vi "AlliGator Logistic Square Gated IRF Characteristics Map.vi"(8 "error in (no error)":errorcluster, 9 "Cursor Names Array":string[](array[string]), 10 "Cursor Positions Array":dbl[](array[numeric]), 11 "AlliGator Internal Variables DVR":refnum<data-value>) -> (0 "error out":errorcluster, 1 "Message":string, 3 "AlliGator Internal Variables DVR":refnum<data-value>)   [LabVIEW 2021, in "AlliGator Scripts.lvlib"]
doc: "Computes the decays of all ROIs and fits them with a logistic square gate model.\n\nSaves the results in an ASCII file."
uses:
  AlliGator Scripts.lvlib
  AlliGator Variables List.ctl
  AlliGator Globals, Variables & Constants.lvlib
  Image/Named ROI Description.ctl
  Image/Image.lvlib
  AlliGator Decay Processing.lvlib
  AlliGator Source Image.lvlib
  <vilib>/vision/Image Controls.llb/IMAQ Image.ctl
  <vilib>/ErrorRing/Error Ring.xnode
  Strings/Strings.lvlib
  Time/Time.lvlib
  AlliGator IRF.lvlib
  Fits/Fit Calculation Method.ctl
  Fits/Fits.lvlib
  Fits/Residual Type.ctl
  Fits/Decay Convolution/Decay Model.ctl
  AlliGator Settings List.ctl
  AlliGator Settings.lvlib
  Fits/Basic Fit Options.ctl
  AlliGator Decay Preprocessing.lvlib
  GUI/GUI.lvlib
  AlliGator Abort.vi
  Fits/Square Pulse/Square Pulse Levels Type.ctl
  Fits/Square Pulse/Square Pulse Options.ctl
  Fits/Non-linear Fitting Algorithm.ctl
  Utilities/Utilities.lvlib
  Fits/IRF(X)PSED/Fit Weights Type.ctl
  Notebook/Notebook.lvlib
  Rich Text Box/Rich Text Box.lvlib
  <vilib>/Utility/error.llb/Error Cluster From Error Code.vi
  <vilib>/Utility/file.llb/Write Delimited Spreadsheet (string).vi
  Variant/Variant to Data/Variant to Data.lvlib
  Fits/Non-linear Fitting Method v2.ctl
  Fits/IRF(X)PSED/Decay Fit Options v2.ctl
  Variant/Variant to Data/Variant to U16.vi
  Phasor/Phasor Reference Series.ctl
  Phasor/Phasor.lvlib
  Phasor/Phasor (g, s).ctl
  Phasor/Calibration Phasor (m, phi).ctl
  AlliGator Data Series Type.ctl
  AlliGator Files.lvlib
  AlliGator Internal Variables v2.ctl
  AlliGator Internal Variables.lvlib
  AlliGator Decay Metadata v3.ctl
  AlliGator Phasor Graph.lvlib
  AlliGator Raw Phasor Plot Data v4.ctl
  AlliGator Baseline Subtraction Method.ctl
  AlliGator Decay Background Subtraction Info.ctl
  Graphs/XY Graph/XY Graph Plot Shift Method.ctl
  Graphs/XY Graph/XY Graph Add-Ons.lvlib
  Graphs/XY Graph/XY Graph Plot Shift Parameters.ctl
  AlliGator Decay Extrapolation Parameters.ctl
  AlliGator FLI Dataset Type.ctl
  Phasor/Phasor Harmonic Data.ctl
  AlliGator Phasor Multi-Harmonic Data.ctl
  AlliGator Phasor Plot.lvlib
  AlliGator Displayed Image.ctl
  Fits/IRF(X)PSED/Decay Fit Parameters & Derived Quantities List.ctl
  Fits/IRF(X)PSED/Decay Fit Parameters In List.ctl
  AlliGator Decay Fit Parameter Constraints 2.ctl
  AlliGator Decay Fit.lvlib
  AlliGator Decay Fit Options & Parameters v2.ctl
  AlliGator Decay Fit Parameter Map.lvlib
  AlliGator Gate Image Set.ctl
  AlliGator Gate Arithmetic.ctl
  AlliGator Dataset Channel.ctl
  AlliGator Dual-Channel Datasets.lvlib
  AlliGator Decay Preprocessing Parameters.ctl
  Phasor/Phasor Standard Deviation Options.ctl
  Phasor/Phasor Calibration Map v2.ctl
  Fits/IRF(X)PSED/MLE Baseline Offset Type.ctl
  AlliGator Parameter Maps Data.ctl
panel:
  # "see the AlliGator License on the block diagram (Ctrl+E or Window:Show Block Diagram)"
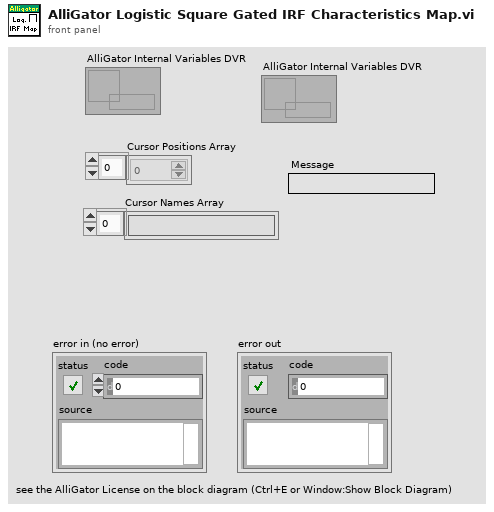
[diagram p1: front panel]
types:
  T1 = typedef "AlliGator Globals, Variables & Constants.lvlib/AlliGator Variables List.ctl" = enum16{"---- GUI ----", "GUI:Initialization Status", "GUI:State Indicators Refnum", "GUI:Original AlliGator Menu Items", "GUI:Current Action Loop State", "GUI:Script in progress", "GUI:Playback", "GUI:Loop Playback", "GUI:Search ROI Used", "GUI:Search ROI", "Decay Graph Max Legend Size", "Intensity Graph Max Legend Size", "Decay Statistics Graph Max Legend Size", "Phasor Graph Max Legend Size", "Phasor Ratio Graph Max Legend Size", "Lifetime Graph Max Legend Size", "---- Files ----", "Files:Export Dataset Frames as Individual Files", "Files:Show Batch Export Help Balloons", "Files:Frames in Dataset", "Files:ptu File Frame Start Indices", "Files:Current Frame in Dataset", "Files:Current Frame Timestamp", "Files:Dataset Loaded", "Files:Dataset Metadata", "Files:Dataset Channel", "Files:Dataset Data Description", "Files:Background Dataset Metadata", "Files:Background Dataset Channel", "Files:Background Dataset Data Description", "Files:Background File Subtraction", "Files:Background File Path", "Files:Background File Pile-up Correction", "Files:Background File Pixel Well Capacity", "Files:Background File Scaling Factor", "Files:Current Dataset Load Settings", "Files:Dataset Path", "Files:ICCD-specific Information", "Files:Macrotime Gate Separation", "------ Python Plugins ------", "Python Plugins:Information", "Python Plugins:Python Session", "Python Plugins:Valid Python Session?", "---- Source Image ----", "Source Image:ROIs", "Source Image:Current ROI", "Source Image:ROI Event Refnum", "X_Source Image Display Range", "X_Source Image Palette Information", "X_Type of Displayed Image", "X_Time Gate Slider", "Source Image:Palette List", "Source Image:Scale", "Source Image:ROI Overlay Color", "Source Image:Overlay to Erase", "Source Image:Is Displayed Image Accumulated", "Source Image:White Light Image Modified", "Source Image:Mask Image Modified", "---- Image Profile Window ----", "Image Profile:Overlay ROI in Source Image", "Image Profile:Window Event Refnum", "Image Profile:IntensityType", "Image Profile:Intensity Average Type", "Image Profile:Intensity-weighted SDV", "Image Profile:Box Profile Type", "Image Profile:Window Open", "Image Profile:Plotted Fit Parameter", "------ Phasor Graph -------", "Phasor Graph:Show Line", "---- Phasor Plot ---", "Phasor Plot:Parameters Changed", "Phasor Plot:FLI Dataset Modified since last Calculation", "Phasor Harmonics Data", "Selected Phasor Harmonics", "Phasor Harmonic Manager Event Refnum", "Phasor Plot:ROIs", "Phasor Plot:Current ROI", "Phasor Plot:ROI Event Refnum", "Phasor Plot:Image Reference Points", "Phasor Plot:Computed", "Phasor Plot:Palette Information", "Phasor Plot:Palette List", "Phasor Plot:Phasor Ratio Palette Information", "Phasor Plot:Phasor Ratio Palette List", "Phasor Plot:Image Scale", "Phasor Plot:Image Overlay to Erase", "Phasor Plot:Image Elements to Update", "Phasor Plot:Current Calculation Parameters", "Phasor Plot:Current Calibration Options", "Phasor Plot:Reset Cumulated Phasor Plot", "Phasor Plot:Reference 1", "Phasor Plot:Lifetime Reference 1", "Phasor Plot:Reference 1 Frequency", "Phasor Plot:Reference 2", "Phasor Plot:Lifetime Reference 2", "Phasor Plot:Reference 2 Frequency", "---- Decay Analysis ----", "Number of Selected Decays to Fit", "LS Fit Results", "LAR Fit Results", "BS Fit Results", "Last Decay Max - Min", "Best Fit Parameters", "Best Fit Parameter Names", "Actual Size X", "Actual Size Y", "Binning X", "Binning Y", "Actual # Gates", "Dataset Number", "Gates to...", "Gates Skipped", "Gates to keep", "Gate Step", "Gate Separation", "Reversed Gates", "Pile-up Correction", "Pixel Well Capacity", "Background Subtracted", "Background Subtraction Method", "Background Definition Range", "Background File (deprecated)", "Number of Dataset Accumulated", "Array of Accumulated Dataset Paths", "Do Averaged Datasets", "Destination File Path", "Process Plot Target", "Use 1/D as Phasor Frequency", "---- Decay Fit Parameter Map -----", "Decay Fit Parameter Map:Palette Information", "Decay Fit Parameter Map:Palette List", "------- Local Decay Window ---------", "Local Decay Graph Window:Event Refnum", "Local Decay Graph Window:Use normalized IRF for convolution", "----- Miscellaneous ----", "Misc:Skippable Dialog Windows Status"}
  T2 = typedef "IMAQ Image.ctl" = refnum<image>
  T3 = typedef "Fits.lvlib/Square Pulse Options.ctl" = cluster{"Method":T4, "# Bins":i32, "Threshold %":dbl, "Center on Midpoint":bool, "Smoothen Plot":bool}
  T4 = typedef "Fits.lvlib/Square Pulse Levels Type.ctl" = enum16{"Mode", "Mean"}
  T5 = typedef "AlliGator Settings.lvlib/AlliGator Settings List.ctl" = enum16{"GUI:Visible Settings Tab", "GUI:Last Run Version", "Source Image:Use Image Histogram for Contrast", "Source Image:Low Count Pixels Rejection Options", "Source Image:High Count Pixels Rejection Options", "Source Image:Use Image Brightness", "Source Image:Blend Overlay with Image Background", "Source Image:Use Fixed ROI Diameter", "Source Image:ROI Diameter", "Source Image:ROI Center Color", "Source Image:Peak Threshold", "Source Image:Intensity Threshold", "Source Image:Image Binning Options", "Source Image:Image Smoothing Options", "Source Image:Image Histogram Active", "Source Image:Invert Binary Mask", "Source Image:Hot Pixel Removal", "Source Image:Overlay Analyzed ROI Center", "Source Image:Auto-Adjust Contrast", "Source Image:Histogram Lower Percentile", "Source Image:Histogram Upper Percentile", "Source Image:Save Source Image", "Source Image:Scale Bar Options", "Source Image:Image Resolution (Pixel Size)", "Source Image:Flatfield Correction", "Source Image:Show Dead Left Columns Correction", "Source Image:Dead Left Columns Correction", "Source Image:Image Pre-Processing Operations Order", "Data Information:Gate Width", "Data Information:Nanotime Gate Separation", "Data Information:Macrotime Gate Separation", "Data Information:Gate Step", "Data Information:# Gates", "Data Information:Gate Image Exposure", "Data Information:Gate Image Integration", "Data Information:Gates to Skip", "Data Information:Gates to Keep", "Data Information:Define Gates to", "Data Information:Channel Name", "Data Information:Available Channel Names", "Data Information:Channel Arithmetic", "Data Information:Background File Subtraction", "Data Information:Background File", "Data Information:Background Scaling Factor", "Data Information:Background Pile-up Correction", "Data Information:Background Pixel Well Capacity", "Data Information:Laser Period", "Data Information:SYNC Period", "Data Information:Pile-up Correction", "Data Information:Pixel Well Capacity", "Data Information:Dataset Scaling Factor", "Fluorescence Decay_Decay Pre-Processing:Reverse Gates", "Fluorescence Decay_Decay Pre-Processing:Verbose Decay Pre-Processing", "Fluorescence Decay_Decay Pre-Processing:Use Decay Pre-Processing", "Fluorescence Decay_Decay Pre-Processing:Background Subtraction", "Fluorescence Decay_Decay Pre-Processing:Background Definition Range", "Fluorescence Decay_Decay Pre-Processing:Baseline Subtraction Method", "Fluorescence Decay_Decay Pre-Processing:Decay Pre-Processing Operations Order", "Fluorescence Decay_Decay Pre-Processing:Smoothing Parameter", "Fluorescence Decay_Decay Pre-Processing:Shift Decay", "Fluorescence Decay_Decay Pre-Processing:Decay Shift Parameters", "Fluorescence Decay_Decay Pre-Processing:Fold Decay", "Fluorescence Decay_Decay Pre-Processing:# Folds", "Fluorescence Decay_Decay Pre-Processing:1-Normalize Decay", "Fluorescence Decay_Decay Pre-Processing:[0-1]-Normalize Decay", "Fluorescence Decay_Decay Pre-Processing:Smoothen Decay", "Fluorescence Decay_Decay Pre-Processing:Extrapolate Decay", "Fluorescence Decay_Decay Pre-Processing:Use Periodicity", "Fluorescence Decay_Decay Pre-Processing:Use Cursors", "Fluorescence Decay_Decay Pre-Processing:Tail Fraction", "Fluorescence Decay_Decay Pre-Processing:Head Fraction", "Fluorescence Decay_Decay Pre-Processing:Additional Points", "Fluorescence Decay_Decay Pre-Processing:Straighten Decay", "Fluorescence Decay_Decay Pre-Processing:Constant Background", "Fluorescence Decay_Decay Pre-Processing:Pixel-Normalize Decay", "Fluorescence Decay_Advanced Analysis:Extract IRF instead of Decay", "Fluorescence Decay_Advanced Analysis:IRF Extraction Options", "Fluorescence Decay_Advanced Analysis:IRF Optimization Options", "Fluorescence Decay_Advanced Analysis:Square Pulse Options", "Fluorescence Decay_Advanced Analysis:IRF Order", "Fluorescence Decay_Advanced Analysis:IRF Time Constants", "Fluorescence Decay_Advanced Analysis:Wavelet Analysis Options", "Fluorescence Decay_Advanced Analysis:Average Lifetime Options", "Fluorescence Decay_Fit Options:Fit Options", "Fluorescence Decay_Fit Options:Use Legacy Fitting Approach", "Fluorescence Decay_Fit Options:Use Data Information Laser Period", "Fluorescence Decay_Fit Parameters:Displayed Fit Parameters", "Fluorescence Decay_Fit Parameters:Fit Parameter Constraints", "Fluorescence Decay_Fit Parameters:Export Tabulated Results", "Fluorescence Decay_Fit Parameters:MLE Baseline Offset Type", "Fluorescence Decay_Fit Parameters:MLE Baseline Offset", "Fluorescence Decay_Fit Parameters:Guess Parameter Names", "Fluorescence Decay_Fit Parameters:Guess Parameter Values", "Fluorescence Decay_Fit Parameters:Guess Parameters Options", "Fluorescence Decay_Styles:Show Last Decay Only", "Fluorescence Decay_Styles:Decay Graph Color Array", "Fluorescence Decay:Decay Graph Active", "Fluorescence Decay Statistics:Min Peak Value", "Fluorescence Decay Statistics:Reject Low Decay Peak Pixels", "Fluorescence Decay Statistics:Reject High Decay Peak Pixels", "Fluorescence Decay Statistics:Max Peak Value", "Time Traces:Use File Timestamp", "Time Traces:Time Step", "Time Traces:Use Intensity Correction File", "Time Traces:Intensity Correction File", "Phasor Plot:Phasor Plot Smoothing Options", "Phasor Plot:Phasor Plot Size", "Phasor Plot:Phasor Plot Graphics Options", "Phasor Plot:Cumulative Phasor Plot", "Phasor Plot:Use Phasor Brightness", "Phasor Plot:Blend Overlay with Phasor Background", "Phasor Plot:Save Phasor Plot", "Phasor Plot:Show References", "Phasor Plot:Phasor Ratio Decay Range", "Phasor Plot:Exponential Fading", "Phasor Plot:Phasor Ratio Reference Colors", "Phasor Plot:Reference Radius", "Phasor Plot:Show Color Map Vertices", "Phasor Plot:Phasor Plot Active", "Phasor Plot:Phasor Ratio Color Map Type", "Phasor Plot:Phasor Ratio Color Map", "Phasor Plot:Phasor Ratio Display Range", "Phasor Plot:Selected Image ROI(s)", "Phasor Plot:All Image ROIs", "Phasor Plot:Selected Phasor Plot ROI(s)", "Phasor Plot:All Phasor Plot ROIs", "Phasor Plot:Phasor Ratio Color-Coded Quantity", "Phasor Plot:Store Phasor Harmonics", "Phasor Plot:Draw Reference Segment", "Phasor Plot:User-Defined Quantity", "Phasor Graph:Phasor Frequency", "Phasor Graph:Phasor Ratio Type", "Phasor Graph:Pixel-level Phasor Computation", "Phasor Graph:Save Phasor Graph", "Phasor Graph:Phasor Graph Active", "Phasor Graph:Phasor SDV Options", "Phasor Calibration:Use Backup Calibration if needed", "Phasor Graph:Define Shortest Lifetime as", "Phasor Calibration:Backup Calibration Type", "Phasor Calibration:Calibration Type", "Phasor Calibration:Calibration Lifetime", "Phasor Calibration:Calibration Map Algorithm", "Single-Exponential Phasor Locus (SEPL):Gate Parameters", "Single-Exponential Phasor Locus (SEPL):User-defined Gate", "Single-Exponential Phasor Locus (SEPL):User-defined IRF", "Single-Exponential Phasor Locus (SEPL):Phasor Parameters", "Single-Exponential Phasor Locus (SEPL):Decay & IRF Parameters", "Single-Exponential Phasor Locus (SEPL):Display Parameters", "Lifetime Analysis:Decay Analysis Parameters", "Lifetime Analysis:Lifetime Map Active", "Plugins:Python Settings", "Miscellaneous:Verbose Mode", "Miscellaneous:Beep after Script", "Miscellaneous:Saved Image File Format", "Miscellaneous:Exported Gate Image Settings", "Miscellaneous:Include Loading in Timing", "Miscellaneous:Verbose Settings Mode", "Miscellaneous:Histogram Options", "Miscellaneous:Beep on Error", "Miscellaneous:# Logical Processors Used", "Miscellaneous:ROI Description Max Characters", "Miscellaneous:Verbose Error Mode", "Miscellaneous:Transparent Mask Color"}
  T6 = typedef "Fits.lvlib/Basic Fit Options.ctl" = cluster{"Fitting Method":T7, "Weighted Fit":bool, "Residual Type":T8, "Compute Parameter Uncertainties":bool, "Fitting Algorithm":T9}
  T7 = typedef "Fits.lvlib/Non-linear Fitting Method v2.ctl" = enum16{"Least Square", "Least Absolute Residual", "Bisquare", "MLE", "-", "Best of All"}
  T8 = typedef "Fits.lvlib/Residual Type.ctl" = enum16{"Standard", "Normalized", "Reduced"}
  T9 = typedef "Fits.lvlib/Non-linear Fitting Algorithm.ctl" = enum16{"Levenberg-Marquardt", "Trust-Region Dogleg"}
  T10 = typedef "Fits.lvlib/Decay Fit Options v2.ctl" = cluster{"Show Fit Residuals":bool, "Fit Model":T11, "Residual Type":T8, "Max Decay Percentile":dbl, "Min Decay Percentile":dbl, "Show Full Decay":bool, "Weights":T12, "Fitting Method":T7, "Compute Parameter Uncertainties":bool, "Periodic Boundaries":bool, "Model Calculation":T13, "Period":dbl[unit], "Termination Criteria":cluster{"Max Iterations":i32, "Max Function Calls":i32, "Max Time":dbl[unit], "Function Tolerance":dbl, "Parameter Tolerance":dbl, "Gradient Tolerance":dbl, "Min Lambda":dbl, "Max Lambda":dbl, "Initial Tick Count":u32}, "Offset Resolution":dbl[unit], "Use Local IRF":bool, "Fitting Algorithm":T9}
  T11 = typedef "Fits.lvlib/Decay Model.ctl" = enum16{"1-Exponential", "2-Exponentials"}
  T12 = typedef "Fits.lvlib/Fit Weights Type.ctl" = enum16{"Unweighted", "1/Variance", "Best of All"}
  T13 = typedef "Fits.lvlib/Fit Calculation Method.ctl" = enum16{"Simulation", "Convolution", "Integration"}
  T14 = typedef "Image.lvlib/Named ROI Description.ctl" = cluster{"ROI Descriptor":T15, "ROI Name":string, "Overlay Color":u32}
  T15 = typedef "ROI Descriptor" = cluster{"Global Rectangle":i32[], "Contours":cluster{"ID":enum32{"External", "Internal"}, "Type":u32, "Coordinates":i32[]}[]}
  T16 = typedef "AlliGator Internal Variables.lvlib/AlliGator Internal Variables v2.ctl" = cluster{"Displayed Image":T2, "White Light Image":T2, "Mask Image":T2, "ROI Mask Image":T2, "Current Dataset Images 1":T17, "Background Dataset Images 1":T17, "Current Dataset Images 2":T17, "Background Dataset Images 2":T17, "Current Dataset Arithmetic Images":T17, "Accumulated Dataset Images 1":T17, "Accumulated Dataset Images 2":T17, "Accumulated Dataset Arithmetic Images":T17, "Phasor Plot Image":T2, "Decay Fit Parameter Map Image":T2, "Single Data Point Path":path, "White Light Image Path":path, "Mask Image Path":path, "Time-Series Folder":path, "[Time-Series Paths]":path[], "Current Dataset":i32, "Single Dataset Type":T18, "Current Folder":string, "AlliGator Data Series Type":T19, "# Datasets":i32, "Dual-Channel Dataset":bool, "Selected Channel Name":string, "Dataset Channel":T20, "Channel Arithmetic":T21, "Dual-Channel Background Dataset":bool, "Background Channel":T20, "Dual-Channel Accumulated Dataset":bool, "Start Time":dbl, "[Time-Series Timestamps]":dbl[], "[Intensity Corrections]":dbl[], "Time Series Script":bool, "Type of Displayed Image":T22, "Gate Image Slide":u16, "# Gates":i32, "ROIs":T14[], "ROI Decay":cluster{"t Array":dbl[], "I Array":dbl[]}, "Valid Decay":bool, "Decay  Metadata":T23, "Reference Decay Plot Name":string, "Reference Decay":cluster{"t Array":dbl[], "I Array":dbl[]}, "Decay Shift Plot":cluster{"Time Stamps":dbl[], "Decay Shifts":dbl[]}, "[Decays Max Values]":sgl[], "[Decays Min Values]":sgl[], "Calibration Phasor":T29, "Calibration Phasor Series":T30, "Phasor Calibration Map":T31, "Calibration Map MD5 Digest":string, "Last Raw Phasor":T32, "Last Calibrated Phasor":T32, "Last Calibrated Phasor SDV":T32, "Phasor Graph:Phasor Plot":cluster{"g Array":dbl[], "s Array":dbl[]}, "Phasor Graph:Phasor SDV Plot":cluster{"g Array":dbl[], "s Array":dbl[]}, "[Phasor Graph:Raw Phasor Plots]":T33[], "Phasor Plot locked to Ref 1":i32, "[Phasor Plot(s) locked to Ref 1]":i32[], "[Phasor Plot(s) locked to Ref 2]":i32[], "[Pixel Phasors]":T32[], "[[Sum Image]]":dbl[][], "[[CSG Phasors]]":csg[][], "[[Valid Pixel?]]":bool[][], "I/m/phi Dataset":cluster{"I/m/phi Dataset?":bool, "Base Frequency":dbl[unit], "Harmonic Orders":u8[]}, "Multi Phasor Plot Data":T35, "Decay Fit Options & Parameters":T37, "Fit Options: Decay Preprocessing Parameters":T41, "Fit Options: Reference Decay":cluster{"t Array":dbl[], "I Array":dbl[]}, "Is Full Image Parameters Map":bool, "Is Single-Pixels Parameters Map":bool, "NLSF Parameters Map X Resolution":i32, "NLSF Parameters Map Y Resolution":i32, "[Single Decay Fit Parameters]":dbl[], "Fit Model":T11, "[[Multiple Decays Fit Parameters]]":dbl[][], "[[Multiple Decays Fit Parameter SDVs]]":dbl[][], "[[IRFs]]":dbl[][], "IRF Array Time Axis":dbl[], "Decay Array Time Axis":dbl[], "[Decay Fit Parameter Names]":T42[], "[[Phasor Ratios]]":dbl[][], "[[Average Lifetimes]]":dbl[][], "Amplitude Weighted Average Lifetime":bool, "[Decay Sum]":dbl[], "Parameter Maps":T43[], "[[User-defined Quantities]]":dbl[][], "User-defined Quantity":string}
  T17 = typedef "AlliGator Internal Variables.lvlib/AlliGator Gate Image Set.ctl" = cluster{"SGL Image Max":T2, "SGL Image Sum":T2, "SGL Gate Images":T2[], "SGL Image Min":T2}
  T18 = typedef "AlliGator Files.lvlib/AlliGator FLI Dataset Type.ctl" = enum16{"HDF5 FLI Dataset", "Gate Image Folder", ".sdt FLI Dataset (Becker & Hickl)", ".ptu FLI Dataset (PicoQuant)", "SS1 FLI Dataset", "SS2 FLI Dataset", "I/m/phi Dataset", ".bin FLI Dataset (PicoQuant Binned)", ".bin FLI Dataset (Piccolo Binned)"}
  T19 = typedef "AlliGator Files.lvlib/AlliGator Data Series Type.ctl" = enum16{"Not a Supported Series", "Gate Images Folder Series", "SwissSPAD 2 Dataset Series", "B&H FLI Dataset Series", "PicoQuant PTU FLI Dataset Series", "PicoQuant BIN FLI Dataset Series", "Piccolo hist BIN FLI Dataset Series", "HDF5 FLI Dataset Series"}
  T20 = typedef "AlliGator Dual-Channel Datasets.lvlib/AlliGator Dataset Channel.ctl" = enum16{"G2", "INT"}
  T21 = typedef "AlliGator Settings.lvlib/AlliGator Gate Arithmetic.ctl" = enum16{"None", "INT-G2", "G2/INT*<INT>", "(1 - G2/INT)*<INT>"}
  T22 = typedef "AlliGator Source Image.lvlib/AlliGator Displayed Image.ctl" = enum16{"Single Gate", "Sum of All Gates", "Max of All Gates", "Min of All Gates", "-", "White Ligth Image", "Mask Image"}
  T23 = typedef "AlliGator Phasor Graph.lvlib/AlliGator Decay Metadata v3.ctl" = cluster{"ROI Descriptor":T15, "ROI Center":cluster{"X":i32, "Y":i32}, "Decay Background Subtraction Info":T24, "Decay Reverted":bool, "Decay Smoothened":bool, "Decay Straightened":bool, "Fitted Tau (Decay Straightening)":dbl, "Decay Shift Parameters":T26, "Decay Shifted":bool, "Decay Extrapolated":bool, "Decay Extrapolation Parameters":T28, "Decay Normalized":bool, "Fold Decay":bool, "# Folds":u32}
  T24 = typedef "AlliGator Decay Analysis.lvlib/AlliGator Decay Preprocessing.lvlib/AlliGator Decay Background Subtraction Info.ctl" = cluster{"Laser Period":dbl[unit], "Gate Duration":dbl[unit], "Baseline Subtraction Method":T25, "Background Definition Range":cluster{"Min Gate":dbl[unit], "Max Gate":dbl[unit]}, "Total Intensity w/o Bkgd Subtraction":dbl, "Bkgd-subtracted Intensity (exp)":dbl, "# Data Points":i32, "Background/Gate":dbl, "Fitted Lifetime":dbl[unit], "Bkgd-subtracted Intensity (theo)":dbl}
  T25 = typedef "AlliGator Decay Analysis.lvlib/AlliGator Decay Preprocessing.lvlib/AlliGator Baseline Subtraction Method.ctl" = enum16{"Mean", "Min", "Square Gated Single-Exponential", "File", "Constant"}
  T26 = typedef "XY Graph Add-Ons.lvlib/XY Graph Plot Shift Parameters.ctl" = cluster{"Type":T27, "Shift":dbl[unit], "Threshold":dbl, "Rotate":bool}
  T27 = typedef "XY Graph Add-Ons.lvlib/XY Graph Plot Shift Method.ctl" = enum16{"Default", "CFD", "Threshold", "Cross-Correlation"}
  T28 = typedef "AlliGator Decay Analysis.lvlib/AlliGator Decay Preprocessing.lvlib/AlliGator Decay Extrapolation Parameters.ctl" = cluster{"Additional Points":u32, "Head Fraction":dbl, "Fitted Tau":dbl, "Use Periodicity":bool, "Use Cursors":bool, "Tail Fraction":dbl}
  T29 = typedef "Phasor.lvlib/Calibration Phasor (m, phi).ctl" = cluster{"m":dbl, "phi":dbl, "Phasor Frequency":dbl[unit], "Reference Lifetime":dbl[unit]}
  T30 = typedef "Phasor.lvlib/Phasor Reference Series.ctl" = cluster{"m Array":dbl[], "phi Array":dbl[], "Phasor Frequency":dbl[unit], "Calibration Lifetime":dbl[unit]}
  T31 = typedef "Phasor.lvlib/Phasor Calibration Map v2.ctl" = cluster{"Phasor Frequency":dbl[unit], "Calibration Lifetime":dbl[unit], "ROI Centers":cluster{"X":i32, "Y":i32}[], "ROI Descriptors":T15[], "Map Resolution X":i32, "Map Resolution Y":i32, "z Array":cdb[]}
  T32 = typedef "Phasor.lvlib/Phasor (g, s).ctl" = cluster{"g":dbl, "s":dbl}
  T33 = typedef "AlliGator Phasor Graph.lvlib/AlliGator Raw Phasor Plot Data v4.ctl" = cluster{"Phasor Plot Name":string, "Raw Phasor Plot":T32[], "Phasor Frequency":dbl[unit], "[Decay Metadata]":T23[], "Raw Phasor Plot SDV":T32[], "Phasor SDV Options":T34, "[Calibration Phasor]":T29[]}
  T34 = typedef "Phasor.lvlib/Phasor Standard Deviation Options.ctl" = cluster{"Compute Estimated SDV":bool, "# Replicas":u32, "Use Estimated Average Phasor":bool}
  T35 = typedef "AlliGator Phasor Plot.lvlib/AlliGator Phasor Multi-Harmonic Data.ctl" = cluster{"Base Frequency":dbl[unit], "# Harmonics":u8, "Harmonic Orders":u8[], "Phasor Plot Settings Checksum":u64, "Phasor Harmonic Data Array":T36[]}
  T36 = typedef "Phasor.lvlib/Phasor Harmonic Data.ctl" = cluster{"Phasor Harmonic Name":string, "Phasor Plot Settings Checksum":u64, "Phasor Frequency":dbl[unit], "Base Frequency":dbl[unit], "Harmonic Order":u8, "Phasor Plot Parameters":string, "Phasor Array [[CSG]]":csg[][], "Dataset File Path":path}
  T37 = typedef "AlliGator Decay Fit Parameter Map.lvlib/AlliGator Decay Fit Options & Parameters v2.ctl" = cluster{"SYNC Period":dbl[unit], "Fit Options":T10, "Fit Parameter Constraints":T38[], "MLE Baseline Offset":dbl, "MLE Baseline Offset Type":T40}
  T38 = typedef "AlliGator Decay Analysis.lvlib/AlliGator Decay Fit.lvlib/AlliGator Decay Fit Parameter Constraints 2.ctl" = cluster{"Fit Parameter":T39, "Min Value":dbl, "Max Value":dbl, "Global":bool, "Used":bool}
  T39 = typedef "Fits.lvlib/Decay Fit Parameters In List.ctl" = enum16{"Offset", "Baseline", "A_1", "tau_1", "A_2", "tau_2"}
  T40 = typedef "Fits.lvlib/MLE Baseline Offset Type.ctl" = enum32{"Absolute", "Percentage"}
  T41 = typedef "AlliGator Decay Analysis.lvlib/AlliGator Decay Preprocessing.lvlib/AlliGator Decay Preprocessing Parameters.ctl" = cluster{"Background Subtraction":bool, "Straighten Decay":bool, "Reverse Gates":bool, "1-Normalized Decay":bool, "Smoothen Decay":bool, "Smoothing Parameter":dbl, "Shift Decay":bool, "Decay Shift Parameters":T26, "Extrapolate Decay":bool, "Additional Points":u32, "Head Fraction":dbl, "Pixel-Normalize Decay":bool, "Use Periodicity":bool, "Use Cursors":bool, "Tail Fraction":dbl, "Use Decay Pre-Processing":bool, "Fold Decay":bool, "# Folds":u32, "[0-1]-Normalized Decay":bool}
  T42 = typedef "Fits.lvlib/Decay Fit Parameters & Derived Quantities List.ctl" = enum16{"Offset", "Baseline", "A_1", "tau_1", "A_2", "tau_2", "<tau>_a", "f1_a", "f2_a", "<tau>_i", "f1_i", "f2_i", "-", "R^2", "Chi^2"}
  T43 = typedef "AlliGator Parameter Maps Data.ctl" = cluster{"Map Set Name":string, "[Parameter Names]":string[], "[[Parameters]]":dbl[][], "[[Parameter SDVs]]":dbl[][], "Decay Array Time Axis":dbl[], "[[IRFs]]":dbl[][], "IRF Array Time Axis":dbl[]}
  T44 = typedef "AlliGator Settings.lvlib/AlliGator Pixel Counts Constraints.ctl" = cluster{"High Count Pixels Rejection Options":T45, "Low Count Pixels Rejection Options":T46}
  T45 = typedef "AlliGator Settings.lvlib/AlliGator High Count Pixels Rejection Options.ctl" = cluster{"Background High Threshold Factor":dbl, "Fixed High Background Threshold":dbl, "Reject High Count Pixels":bool, "High Percentile":dbl}
  T46 = typedef "AlliGator Settings.lvlib/AlliGator Low Count Pixels Rejection Options.ctl" = cluster{"Background Low Threshold Factor":dbl, "Fixed Low Background Threshold":dbl, "Reject Low Count Pixels":bool, "Low Percentile":dbl}
  T47 = cluster{"Decay Peak Constraint":bool, "Min":dbl, "Max":dbl}
  T48 = typedef "Rich Text Box.lvlib/Text Formatting.ctl" = cluster{"Font":string, "Text Color":T49, "Text Background Color":T49, "Text Style":enum16{"Regular", "Bold", "Italic", "Underline", "Strikeout"}, "Font Size (Points)":dbl, "Text Alignment":i32}
  T49 = typedef "Rich Text Box.lvlib/Text Colors.ctl" = enum16{"Unchanged", "Black", "Blue", "Brown", "Gray", "Green", "Orange", "Pink", "Red", "White"}
  T50 = cluster{"t Axis":dbl[], "ROI Intensity Array":dbl[]}
  T51 = typedef "Fits.lvlib/Non-linear Fit Output v3.ctl" = cluster{"best nonlinear fit":dbl[], "best fit parameters":dbl[], "R^2":dbl, "RMSE":dbl, "error out":errorcluster, "Fitting Method":T52, "number of function calls":i32, "number of iterations":i32, "covariance":T53, "Chi 2":dbl, "DOF":i32, "Fit Convergence Criterion":T54, "Fitting Algorithm":T9, "Weighted Fit":bool, "Gradient":dbl, "|Delta Chi 2|":dbl, "|Delta Chi 2|/Chi 2":dbl, "Max |Delta a| /|a|":dbl, "Lambda":dbl, "RSS":dbl, "AIC":dbl, "BIC":dbl, "Max number of function calls":i32, "Max number of iterations":i32, "IRF":T55, "IRF Normalization Factor":dbl, "Decay Normalization Factor":dbl}
  T52 = typedef "Fits.lvlib/Nonlinear Fit Method.ctl" = enum16{"Least Square", "Least Absolute Residual", "Bisquare", "MLE"}
  T53 = typedef "NI_Matrix.lvlib/RealMatrix.ctl" = dbl[][]
  T54 = typedef "Fits.lvlib/Convergence Criteria.ctl" = enum16{"Continue", "Tolerances Exceeded", "Max Time Exceeded", "Max Iterations Exceeded", "Max Function Evaluations Exceeded", "Scale Range Exceeded"}
  T55 = typedef "XY Graph Add-Ons.lvlib/XY Plot Data.ctl" = cluster{"X Array":dbl[], "Y Array":dbl[]}
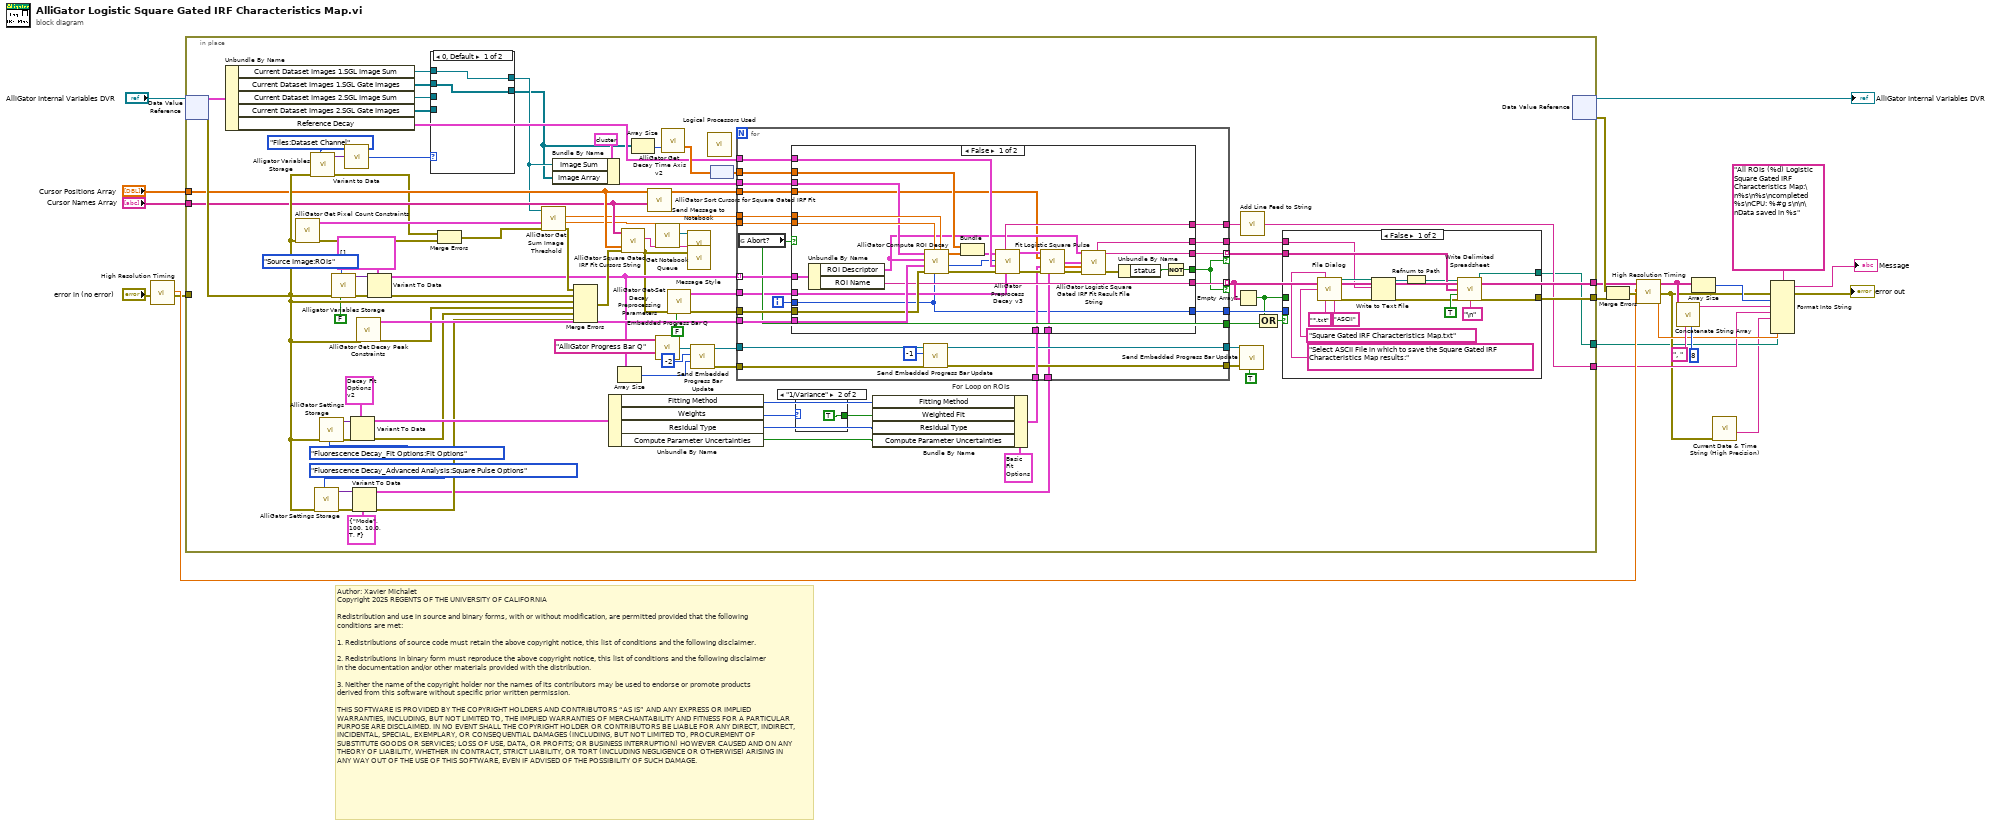
[diagram p0: block diagram]
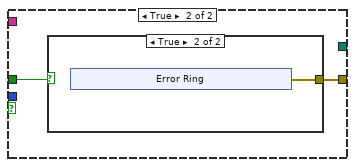
[diagram p4: hidden frame]
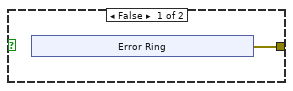
[diagram p5: hidden frame]
diagram:
  # "Author: Xavier Michalet\nCopyright 2025 REGENTS OF THE UNIVERSITY OF CALIFORNIA\n\nRedistribution and use in source and binary forms, with or without modification, are permitted provided that the following conditions are met:\n\n1. Redistributions of source code must retain the above copyright notice, this list of conditions and the following disclaimer.\n\n2. Redistributions in binary form must reproduce the above copyright notice, this list of conditions and the following disclaimer in the documentation and/or other materials provided with the distribution.\n\n3. Neither the name of the copyright holder nor the names of its contributors may be used to endorse or promote products derived from this software without specific prior written permission.\n\nTHIS SOFTWARE IS PROVIDED BY THE COPYRIGHT HOLDERS AND CONTRIBUTORS “AS IS” AND ANY EXPRESS OR IMPLIED WARRANTIES, INCLUDING, BUT NOT LIMITED TO, THE IMPLIED WARRANTIES OF MERCHANTABILITY AND FITNESS FOR A PARTICULAR PURPOSE ARE DISCLAIMED. IN NO EVENT SHALL THE COPYRIGHT HOLDER OR CONTRIBUTORS BE LIABLE FOR ANY DIRECT, INDIRECT, INCIDENTAL, SPECIAL, EXEMPLARY, OR CONSEQUENTIAL DAMAGES (INCLUDING, BUT NOT LIMITED TO, PROCUREMENT OF SUBSTITUTE GOODS OR SERVICES; LOSS OF USE, DATA, OR PROFITS; OR BUSINESS INTERRUPTION) HOWEVER CAUSED AND ON ANY THEORY OF LIABILITY, WHETHER IN CONTRACT, STRICT LIABILITY, OR TORT (INCLUDING NEGLIGENCE OR OTHERWISE) ARISING IN ANY WAY OUT OF THE USE OF THIS SOFTWARE, EVEN IF ADVISED OF THE POSSIBILITY OF SUCH DAMAGE."
  n1 = call "High Resolution Timing.vi"("Error In"="error in (no error)") -> ("elapsed (relative) seconds"=w14:dbl, "Error Out"=w9:errorcluster)  [unwired: 16 in, 1 out]
  n2 = in-place {
    in-place-border: [w104] -> w19
    in-place-border: [w103] -> w11
    in-place-border: w9 -> [_]
    in-place-border: [w101] -> w8
    in-place-border: "Cursor Positions Array" -> [w100]
    in-place-border: "Cursor Names Array" -> [w99]
    in-place-border: [w98] -> w4
    n3 = in-place-dvr #1("AlliGator Internal Variables DVR") -> (w105:T16, w102:errorcluster)
    n4 = Unbundle By Name(w105) -> ("Current Dataset Images 1.SGL Image Sum"=w38:T2, "Current Dataset Images 1.SGL Gate Images"=w39:T2[], "Current Dataset Images 2.SGL Image Sum"=w34:T2, "Current Dataset Images 2.SGL Gate Images"=w35:T2[], "Reference Decay"=w83:cluster{"t Array":dbl[], "I Array":dbl[]})
    n5 = call "AlliGator Get Pixel Count Constraints.vi"("error in (no error)"=w102) -> ("error out"=w91:errorcluster, "Pixel Count Constraints"=w92:T44)  [unwired: 9 in]
    n6 = call "Alligator Variables Storage.vi"("AlliGator Variable"=AlliGator_Variables_List."Files:Dataset Channel" ("Alligator Variable"), "Error In"=w102) -> ("Error Out"=w25:errorcluster, "Data out"=w27:variant)  [unwired: 7 in, 1 out]
    n7 = call "AlliGator Settings Storage.vi"("AlliGator Settings List"=AlliGator_Settings_List."Fluorescence Decay_Advanced Analysis:Square Pulse Options", "Error In"=w102) -> ("Error Out"=w49:errorcluster, "Variant Data out"=w50:variant)  [unwired: 8 in]
    n8 = call "AlliGator Settings Storage.vi"("AlliGator Settings List"=AlliGator_Settings_List."Fluorescence Decay_Fit Options:Fit Options", "Error In"=w102) -> ("Error Out"=w66:errorcluster, "Variant Data out"=w64:variant)  [unwired: 8 in]
    n9 = call "Alligator Variables Storage.vi"("Get(F)/Set"=FALSE, "AlliGator Variable"=AlliGator_Variables_List."Source Image:ROIs" ("Alligator Variable"), "Error In"=w102) -> ("Error Out"=w95:errorcluster, "Data out"=w96:variant)  [unwired: 6 in, 1 out]
    n10 = call-poly "Variant to Data.vi"("Variant"=w27) -> ("U16 Value"=w24:u16)  [unwired: 8 in]
    n11 = Variant To Data(error in=w66, type=T10 {"Show Fit Residuals"=TRUE, "Fit Model"=enum."1-Exponential", "Residual Type"=enum."Standard", "Max Decay Percentile"=0.0, "Min Decay Percentile"=0.0, "Show Full Decay"=TRUE, "Weights"=enum."Unweighted", "Fitting Method"=enum."Least Square", "Compute Parameter Uncertainties"=TRUE, "Periodic Boundaries"=TRUE, "Model Calculation"=enum."Simulation", "Period"=1.2500000000000001e-08, "Termination Criteria"={"Max Iterations"=1000, "Max Function Calls"=0, "Max Time"=1000.0, "Function Tolerance"=1e-06, "Parameter Tolerance"=1e-06, "Gradient Tolerance"=0.0, "Min Lambda"=1e-06, "Max Lambda"=1e-06, "Initial Tick Count"=0}, "Offset Resolution"=1.2500000000000001e-08, "Use Local IRF"=TRUE, "Fitting Algorithm"=enum."Levenberg-Marquardt"} ("Fit Options"), Variant=w64) -> (data=w67:T10, error out=w63:errorcluster)
    n12 = Variant To Data(error in=w49, type=T3 {"Method"=enum."Mode", "# Bins"=100, "Threshold %"=10.0, "Center on Midpoint"=TRUE, "Smoothen Plot"=FALSE} ("Square Pulse Options"), Variant=w50) -> (data=w45:T3, error out=w46:errorcluster)
    n13 = call "AlliGator Get Decay Peak Constraints.vi"("error in (no error)"=w102) -> ("Error Out"=w76:errorcluster, "Decay Peak Constraints"=w87:T47)  [unwired: 9 in]
    n14 = Variant To Data(error in=w95, type=T14[] [] ("Stored ROIs in"), Variant=w96) -> (data=w53:T14[], error out=w90:errorcluster)
    n15 = case shown="0, Default" w24 {
      tunnel: [w107 w109] -> w36
      tunnel: w35 -> [_ w109]
      tunnel: [w106 w108] -> w37
      tunnel: w34 -> [_ w108]
      tunnel: w39 -> [w107 _]
      tunnel: w38 -> [w106 _]
      frame 0, Default {
      }
      frame 1 {
      }
    }
    n16 = Merge Errors(w25, w91) -> (w26:errorcluster)
    n17 = call "AlliGator Get Sum Image Threshold.vi"("error in (no error)"=w26, "Pixel Counts Constraints"=w92, "Image in"=w37) -> ("error out"=w78:errorcluster, "Pixel Threshold Low"=w88:sgl, "Pixel Threshold High"=w89:sgl)  [unwired: 2 in, 4 out]
    n18 = Bundle By Name(cluster=cluster{"Image Sum":T2, "Image Array":T2[]} {"Image Sum"=refnum, "Image Array"=[]} ("Images"), "Image Sum"=w37, "Image Array"=w36) -> (w86:cluster{"Image Sum":T2, "Image Array":T2[]})
    n19 = Merge Errors(w78, w90, w102, w76, w63, w46) -> (w73:errorcluster)
    n20 = Unbundle By Name(w67) -> ("Fitting Method"=w68:T7, "Weights"=w42:T12, "Residual Type"=w69:T8, "Compute Parameter Uncertainties"=w70:bool)
    n21 = Array Size(array=w53) -> (size(s)=w52:i32)
    n22 = call "AlliGator Square Gated IRF Fit Cursors String.vi"("Error In"=w73, "Cursor Positions Array"=w100, "Cursor Names Array"=w99) -> ("Error Out"=w31:errorcluster, "Message"=w30:string)  [unwired: 7 in]
    n23 = Array Size(array=w36) -> (size(s)=w85:i32)
    n24 = call "AlliGator Sort Cursors for Square Gated IRF Fit.vi"("Cursor Name Array in"=w99, "Cursor Position Array in"=w100) -> ()  [unwired: 8 in, 2 out]
    n25 = call "Get Notebook Queue.vi"() -> ("Notebook Queue"=w32:refnum<queue>)  [unwired: 9 in]
    n26 = call "Embedded Progress Bar Q.vi"("Progress Bar Queue Name"="AlliGator Progress Bar Q") -> ("Progress Bar Queue"=w59:refnum<queue>)  [unwired: 6 in]
    n27 = call "AlliGator Get Decay Time Axis v2.vi"("Number of Gates"=w85) -> ("t Array"=w84:dbl[unit][])  [unwired: 14 in]
    n28 = call "AlliGator Get-Set Decay Preprocessing Parameters.vi"("Get (F)/Set"=FALSE, "Error In"=w31) -> ("Error Out"=w61:errorcluster, "Decay Preprocessing Parameters out"=w43:T41)  [unwired: 8 in]
    n29 = call "Message Style.vi"() -> ("Message Formatting"=w33:T48)
    n30 = call "Send Message to Notebook.vi"("Text Formatting"=w33, "Error In"=w31, "Message"=w30, "Notebook Queue"=w32) -> ()  [unwired: 4 in, 2 out]
    n31 = call "Send Embedded Progress Bar Update.vi"("Max Iterations N"=w52, "Current Iteration i (i or -1: standard or || iteration; 0 or -2: first standard or || iteration)"=-2 ("Current Iteration i (i or -1: standard or || iteration; 0 or -2: first standard or || iteration)"), "Progress Bar Queue in"=w59) -> ("Error Out"=w57:errorcluster, "Progress Bar Queue out"=w58:refnum<queue>)  [unwired: 7 in]
    n32 = call "Logical Processors Used.vi"() -> ()  [unwired: 6 in, 1 out]
    n33 = node(w84) -> (w77:dbl[])
    n34 = case shown="\"1/Variance\"" w42 {
      tunnel: [_ TRUE ("Weighted Fit")] -> w41
      frame "Unweighted", Default {
      }
      frame "1/Variance" {
      }
    }
    n35 = Bundle By Name(cluster=T6 {"Fitting Method"=enum."Least Square", "Weighted Fit"=FALSE, "Residual Type"=enum."Standard", "Compute Parameter Uncertainties"=FALSE, "Fitting Algorithm"=enum."Levenberg-Marquardt"} ("Basic Fit Options"), "Fitting Method"=w68, "Weighted Fit"=w41, "Residual Type"=w69, "Compute Parameter Uncertainties"=w70) -> (w62:T6)
    n36 = for "For Loop on ROIs" {
      tunnel: w53 -> [w162] mode=indexing
      tunnel: w89 -> [w161]
      tunnel: w88 -> [w160]
      tunnel: w86 -> [w159]
      tunnel: w87 -> [w158]
      tunnel: [w142] -> w82
      tunnel: w77 -> [w154]
      tunnel: w83 -> [w155]
      tunnel: [w138] -> w81
      tunnel: [w156] -> w103 mode=indexing if=w151
      tunnel: w61 -> [w157]
      tunnel: [w153] -> w79
      tunnel: w100 -> [w149]
      tunnel: [w152] -> w75 mode=indexing if=w151
      tunnel: [w150] -> w74
      tunnel: w62 -> [w148]
      tunnel: w58 -> [w147]
      tunnel: w57 -> [w146]
      tunnel: [w145] -> w56
      tunnel: [w144] -> w55
      tunnel: w45 -> [w141]
      tunnel: w43 -> [w140]
      i -> [w139]
      n37 = global read "AlliGator Abort.vi" "Abort?"() -> (w142:bool)
      n38 = case shown="False" w142 {
        tunnel: w162 -> [w192 _]
        tunnel: w161 -> [w191 _]
        tunnel: w160 -> [w190 _]
        tunnel: w159 -> [w189 _]
        tunnel: w158 -> [w188 _]
        tunnel: w157 -> [w187 _]
        tunnel: [w186 _] -> w156
        tunnel: w155 -> [w184 _]
        tunnel: w154 -> [w182 _]
        tunnel: [w179 _] -> w153
        tunnel: [w173 _] -> w152
        tunnel: [w172 _] -> w151
        tunnel: [w170 _] -> w150
        tunnel: w149 -> [w169 _]
        tunnel: w148 -> [w168 _]
        tunnel: w141 -> [w165 _]
        tunnel: w140 -> [w164 _]
        tunnel: w139 -> [w163 _]
        tunnel: [w163 _] -> w138
        frame False {
          n39 = Unbundle By Name(w192) -> ("ROI Descriptor"=w171:T15, "ROI Name"=w186:string)
          n40 = call "AlliGator Compute ROI Decay.vi"("Pixel Threshold High"=w191, "Loop ID"=w163, "Pixel Threshold Low"=w190, "error in (no error)"=w187, "Decay Peak  Constraints"=w188, "ROI Descriptor"=w171, "Images"=w189) -> ("error out"=w183:errorcluster, "# Valid Pixels"=w166:i32, "Decay Points"=w181:dbl[])  [unwired: 2 out]
          n41 = Bundle(w182, "Decay Points"=w181) -> (w180:cluster{dbl[], "Decay Points":dbl[]})  [unwired: 1 in]
          n42 = call "AlliGator Preprocess Decay v3.vi"("Decay Preprocessing Parameters"=w164, "Error In"=w183, "Time-Gated Reference Decay"=w184, "# Pixels"=w166, "Decay (in)"=w180) -> ("Error Out"=w178:errorcluster, "Decay (out)"=w177:T50, "Message"=w179:string)  [unwired: 3 in, 1 out]
          n43 = call "Fit Logistic Square Pulse.vi"("Decay"=w177, "Boundaries"=w169, "Basic Fit Options"=w168, "error in (no error)"=w178, "Square Pulse Options"=w165) -> ("Fit Output"=w167:T51, "Delta Best Fit Parameters"=w174:dbl[], "error out"=w176:errorcluster)  [unwired: 6 in, 2 out]
          n44 = call "AlliGator Logistic Square Gated IRF Fit Result File String.vi"("error in (no error)"=w176, "Delta Best Fit Parameters"=w174, "Fit Output"=w167, "ROI Descriptor"=w171) -> ("error out"=w175:errorcluster, "Result String"=w173:string, "Header String"=w170:string)  [unwired: 5 in]
          n45 = Unbundle By Name(w175) -> ("status"=w185:bool)
          n46 = Not(x=w185) -> (.not. x?=w172:bool)
        }
        frame True {
        }
      }
      n47 = call "Send Embedded Progress Bar Update.vi"("Error In"=w146, "Current Iteration i (i or -1: standard or || iteration; 0 or -2: first standard or || iteration)"=-1 ("Current Iteration i (i or -1: standard or || iteration; 0 or -2: first standard or || iteration)"), "Progress Bar Queue in"=w147) -> ("Error Out"=w144:errorcluster, "Progress Bar Queue out"=w145:refnum<queue>)  [unwired: 7 in]
    }
    n48 = Empty Array?(array=w103) -> (empty?=w29:bool)
    n49 = call "Send Embedded Progress Bar Update.vi"("Stop Progress Bar (F)"=TRUE ("Hide Progress Bar (F)"), "Error In"=w55, "Progress Bar Queue in"=w56) -> ()  [unwired: 7 in, 2 out]
    n50 = call "Add Line Feed to String.vi"("String"=w79) -> ("String\\n"=w101:string)  [unwired: 8 in]
    n51 = Compound Arithmetic op=OR(w29, w82) -> (w80:bool)
    n52 = case shown="False" w80 {
      tunnel: [w115 w127] -> w104
      tunnel: w81 -> [_ _]
      tunnel: w75 -> [w118 _]
      tunnel: w74 -> [w112 _]
      tunnel: [w111 _] -> w98
      tunnel: w29 -> [_ w126]
      frame False {
        n53 = call "File Dialog"("prompt"="Select ASCII File in which to save the Square Gated IRF Characteristics Map results:" ("prompt (Choose or enter file path)"), "default name"="Square Gated IRF Characteristics Map.txt", "pattern (all files)"="*.txt", "pattern label"="ASCII") -> ("selected path"=w120:path, "error out"=w125:errorcluster)  [unwired: 8 in, 2 out]
        n54 = Write to Text File(file (use dialog)=w120, text=w112, error in=w125) -> (refnum out=w114:refnum<file>, error out=w116:errorcluster)  [unwired: 1 in, 1 out]
        n55 = Refnum to Path(1:w114) -> (0:w113:path)
        n56 = call-poly <vilib>:"Write Delimited Spreadsheet.vi"("file path (dialog if empty)"=w113, "1D data"=w118, "append to file? (new file:F)"=TRUE, "error in (no error)"=w116, "delimiter (\\t)"="\n" ("delimiter (\\t)")) -> ("new file path (Not A Path if cancelled)"=w111:path, "error out"=w115:errorcluster)  [unwired: 9 in]
      }
      frame True {
        n57 = case shown="True" w126 {
          tunnel: [w128 w133] -> w127
          frame False {
            n58 = xnode "Error Ring"() -> ("error out"=w128:errorcluster)
          }
          frame True {
            n59 = xnode "Error Ring"() -> ("error out"=w133:errorcluster)
          }
        }
      }
    }
    n60 = in-place-dvr #1() -> (→"AlliGator Internal Variables DVR":refnum<data-value>, w20:errorcluster)  [unwired: 1 in]
  }
  n61 = Merge Errors(w20, w19) -> (w16:errorcluster)
  n62 = call "High Resolution Timing.vi"("relative seconds (NaN)"=w14, "Error In"=w16) -> ("elapsed (relative) seconds"=w13:dbl, "Error Out"=w7:errorcluster)  [unwired: 15 in, 1 out]
  n63 = call "Concatenate String Array.vi"("Max Number of Elements (None: -1)"=8 ("Max Number of Elements (None: 1)"), "Separator (TAB)"=", ", "String Array"=w11) -> ("Formatted String"=w12:string)  [unwired: 8 in]
  n64 = Array Size(array=w11) -> (size(s)=w10:i32)
  n65 = call "Current Date & Time String (High Precision).vi"("Error In"=w7) -> ("on <Date> at <Time>"=w1:string)  [unwired: 7 in, 3 out]
  n66 = Format Into String(format string="All ROIs (%d) Logistic Square Gated IRF Characteristics Map:\n%s\n%s\ncompleted %s\nCPU: %#g s\n\n\nData saved in %s", error in=w7, w10, w12, w8, w1, w13, w4) -> (resulting string=→"Message":string, error out=→"error out":errorcluster)  [unwired: 1 in]
